vi "epoll_ctl.vi"(8 "error in":errorcluster, 11 "epoll in":refnum<class "epoll.lvclass">) -> (0 "error out":errorcluster, 3 "epoll out":refnum<class "epoll.lvclass">)   [LabVIEW 2019, in "PCANBasic.lvlib" / "epoll.lvclass"]
doc: "This file includes code from the LinuxRT-IPC project (Apache License 2.0) https://github.com/NISystemsEngineering/LinuxRT-IPC\n\nControl interface for an epoll descriptor\n\nThis system call performs control operations on the epoll(7) instance referred to by the file descriptor epfd. It requests that the operation op be performed for the target file descriptor, fd."
uses:
  epoll.lvclass
  epoll.lvclass/epoll.ctl
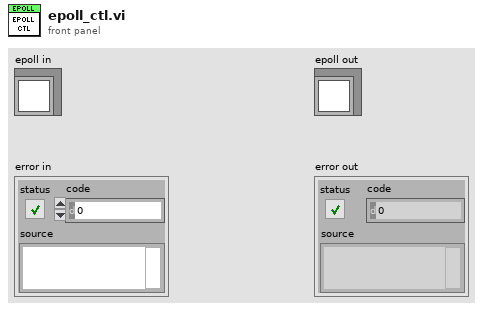
[diagram p1: front panel]
types:
  T1 = enum16{"unspecified", "close", "epoll_create", "epoll_ctl", "epoll_wait"}
  T2 = enum16{"NO ERROR", "EPERM", "ENOENT", "ESRCH", "EINTR", "EIO", "ENXIO", "E2BIG", "ENOEXEC", "EBADF", "ECHILD", "EAGAIN", "ENOMEM", "EACCES", "EFAULT", "ENOTBLK", "EBUSY", "EEXIST", "EXDEV", "ENODEV", "ENOTDIR", "EISDIR", "EINVAL", "ENFILE", "EMFILE", "ENOTTY", "ETXTBSY", "EFBIG", "ENOSPC", "ESPIPE", "EROFS", "EMLINK", "EPIPE", "EDOM", "ERANGE", "EDADLK", "ENAMETOOLONG", "ENOLCK", "ENOSYS", "ENOTEMPTY", "ELOOP", "EWOULDBLOCK", "ENOMSG", "EIDRM", "ECHRNG", "EL2NSYNC", "EL3HLT", "EL3RST", "ELNRNG", "EUNATCH", "ENOCSI", "EL2HLT", "EBADE", "EBADR", "EXFULL", "ENOANO", "EBADRQC", "EBADSLT", "EDEADLOCK", "EBFONT", "ENOSTR", "ENODATA", "ETIME", "ENOSR", "ENONET", "ENOPKG", "EREMOTE", "ENOLINK", "EADV", "ESRMNT", "ECOMM", "EPROTO", "EMULTIHOP", "EDOTDOT", "EBADMSG", "EOVERFLOW", "ENOTUNIQ", "EBADFD", "EREMCHG", "ELIBACC", "ELIBBAD", "ELIBSCN", "ELIBMAX", "ELIBEXEC", "ELISEQ", "ERESTART", "ESTRPIPE", "EUSERS", "ENOTSOCK", "EDESTADDRREQ", "EMSGSIZE", "EPROTOTYPE", "ENOPROTOOPT", "EPROTONOSUPPORT", "ESOCKTNOSUPPORT", "EOPNOTSUPP", "EPFNOSUPPORT", "EAFNOSUPPORT", "EADDRINUSE", "EADDRNOTAVAIL", "ENETDOWN", "ENETUNREACH", "ENETRESET", "ECONNABORTED", "ECONNRESET", "ENOBUFS", "EISCONN", "ENOTCONN", "ESHUTDOWN", "ETOOMANYREFS", "ETIMEDOUT", "ECONNREFUSED", "EHOSTDOWN", "EHOSTUNREACH", "EALREADY", "EINPROGRESS", "ESTALE", "EUCLEAN", "ENOTNAM", "ENAVAIL", "EISNAM", "EREMOTEIO", "EDQUOT", "ENOMEDIUM", "EMEDIUMTYPE", "ECANCELED", "ENOKEY", "EKEYEXPIRED", "EKEYREVOKED", "EKEYREJECTED", "EOWNERDEAD", "ENOTRECOVERABLE", "ERFKILL", "EHWPOISON", "UNDEFINED"}
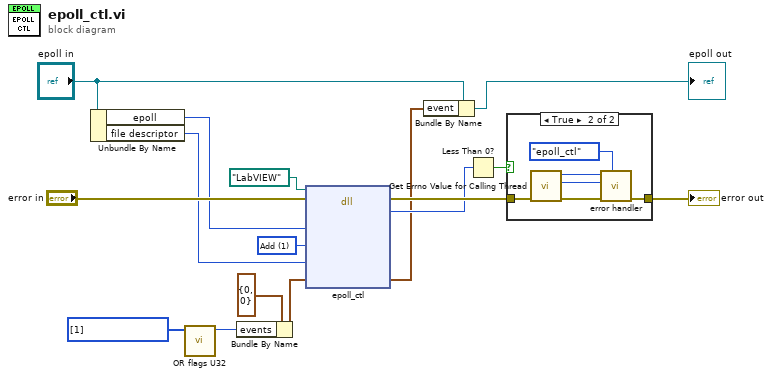
[diagram p0: block diagram]
diagram:
  w7 = u32[] [1] items=["EPOLLIN"=1, "EPOLLPRI"=2, "EPOLLOUT"=4, "EPOLLERR"=8, "EPOLLHUP"=16, "EPOLLRDNORM"=64, "EPOLLRDBAND"=128, "EPOLLWRNORM"=256, "EPOLLWRBAND"=512, "EPOLLMSG"=1024, "EPOLLRDHUP"=8192, "EPOLLWAKEUP"=536870912, "EPOLLONESHOT"=1073741824, "EPOLLET"=2147483648] ("epoll events (default: none)")
  w10 = u32 1 items=["Add"=1, "Delete"=2, "Modify"=3] ("operation")
  n1 = Unbundle By Name("epoll in") -> ("epoll"=w6:i32, "file descriptor"=w5:i32)
  n2 = call "OR flags U32.vi"("flags"=w7) -> ("OR'ed flags"=w9:u32)  [unwired: 10 in]
  n3 = Bundle By Name(cluster=cluster{"events":u32, "data":u64} {"events"=0, "data"=0} ("event"), "events"=w9) -> (w8:cluster{"events":u32, "data":u64})
  n4 = dll-call lib="LabVIEW" fn="epoll_ctl"(path in=path "LabVIEW", error in="error in", "epfd"=w6, "operation"=w10, "fd"=w5, "event"=w8) -> (error out=w15:errorcluster, "return"=w11:i32, "event"=w2:cluster{"events":u32, "data":u64})  [unwired: 4 in, 1 out]
  n5 = Bundle By Name(cluster="epoll in", "event"=w2) -> (→"epoll out":refnum<class "epoll.lvclass">)
  n6 = Less Than 0?(x=w11) -> (x < 0?=w13:bool)
  n7 = case shown="True" w13 {
    tunnel: w15 -> [w17 w23]
    tunnel: [w17 w22] -> w14
    frame False {
    }
    frame True {
      n8 = call "Get Errno Value for Calling Thread.vi"("error in"=w23) -> ("error out"=w20:errorcluster, "errno number"=w19:i32, "errno"=w21:T2)  [unwired: 8 in]
      n9 = call "error handler.vi"("function (unspecified)"=T1."epoll_ctl", "error in"=w20, "errno number"=w19, "errno"=w21) -> ("error out"=w22:errorcluster)  [unwired: 7 in]
    }
  }
  "error out" <- w14
